vi "prepare_experiment.vi"() -> (0 "command out":string)   [LabVIEW 2009]
uses:
  visexpman_variables.vi
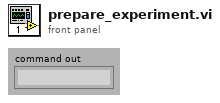
[diagram p1: front panel]
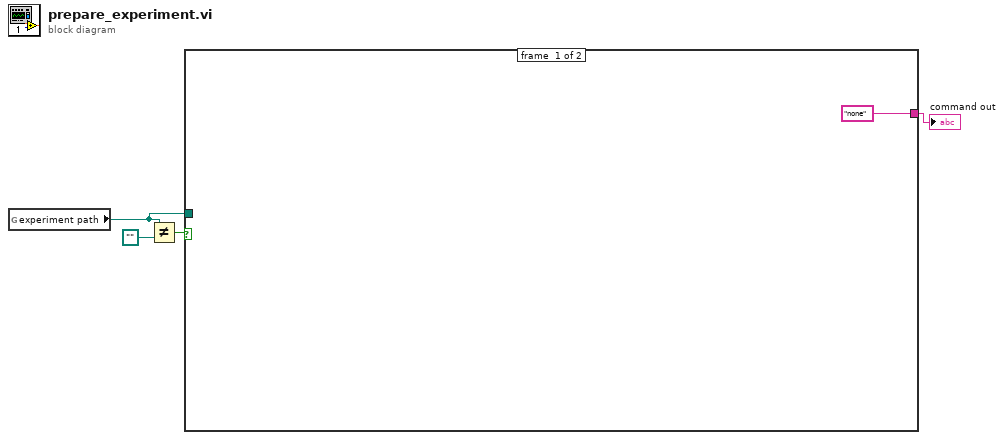
[diagram p0: block diagram]
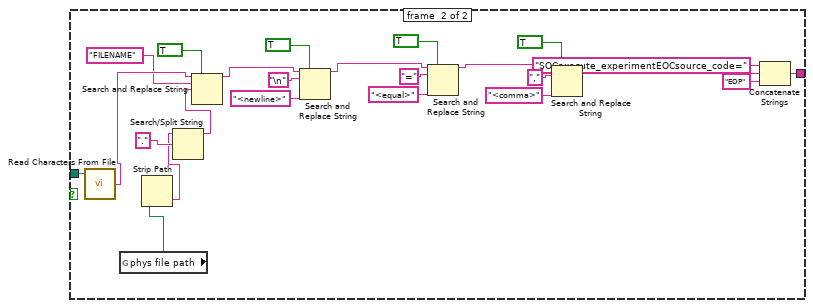
[diagram p2: hidden frame]
diagram:
  n1 = global read "visexpman_variables.vi" "experiment path"() -> (w3:path)
  n2 = Not Equal?(x=w3, y=path "") -> (x != y?=w2:bool)
  n3 = case shown="True" w2 {
    tunnel: w3 -> [_ w27]
    tunnel: ["none" w26] -> w1
    frame #0 {
    }
    frame #1 {
      n4 = call <vilib>:"Read Characters From File.vi"("file path (dialog if empty)"=w27) -> ("character string"=w12:string)  [unwired: 5 in, 3 out]
      n5 = global read "visexpman_variables.vi" "phys file path"() -> (w9:path)
      n6 = Strip Path(path=w9) -> (name=w7:string)  [unwired: 1 out]
      n7 = Search/Split String(string=w7, search string/char (-)="." ("string")) -> (substring before match=w6:string)  [unwired: 1 in, 2 out]
      n8 = Search and Replace String(replace all?=TRUE ("replace all? (F)"), input string=w12, search string="FILENAME" ("replace string (\"\")"), replace string=w6) -> (result string=w11:string)  [unwired: 4 in, 3 out]
      n9 = Search and Replace String(replace all?=TRUE ("replace all? (F)"), input string=w11, search string="\n", replace string="<newline>" ("replace string (\"\")")) -> (result string=w15:string)  [unwired: 4 in, 3 out]
      n10 = Search and Replace String(replace all?=TRUE ("replace all? (F)"), input string=w15, search string="=", replace string="<equal>" ("replace string (\"\")")) -> (result string=w14:string)  [unwired: 4 in, 3 out]
      n11 = Search and Replace String(replace all?=TRUE ("replace all? (F)"), input string=w14, search string=",", replace string="<comma>" ("replace string (\"\")")) -> (result string=w25:string)  [unwired: 4 in, 3 out]
      n12 = Concatenate Strings("SOCexecute_experimentEOCsource_code=" ("string"), w25, "EOP" ("string")) -> (w26:string)
    }
  }
  "command out" <- w1
